vi "Initialize.vi"(8 "error in (no error)":errorcluster, 10 "Laser Configuration":T1, 11 "Laser in":refnum<class "Laser.lvclass">) -> (0 "error out":errorcluster, 3 "Laser out":refnum<class "Laser.lvclass">)   [LabVIEW 2023, in "Laser.lvlib" / "Laser.lvclass"]
uses:
  Laser.lvclass
  Resources/Type Defs/Laser Configuration.ctl
  Laser.lvclass/Laser.ctl
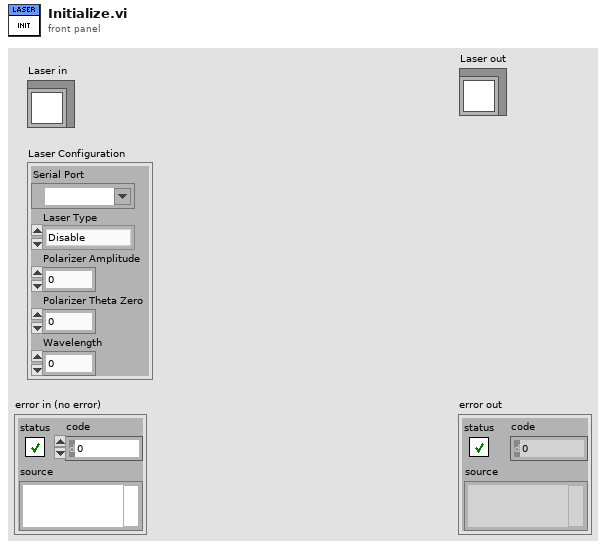
[diagram p1: front panel]
types:
  T1 = typedef "Laser Configuration.ctl" = cluster{"Serial Port":refnum<visa-resource-name>, "Laser Type":enum16{"Disable", "Laser Quantum", "Coherent OBIS", "PRM1-Z8", "Coherent HOPS"}, "Polarizer Amplitude":dbl, "Polarizer Theta Zero":dbl, "Wavelength":u16}
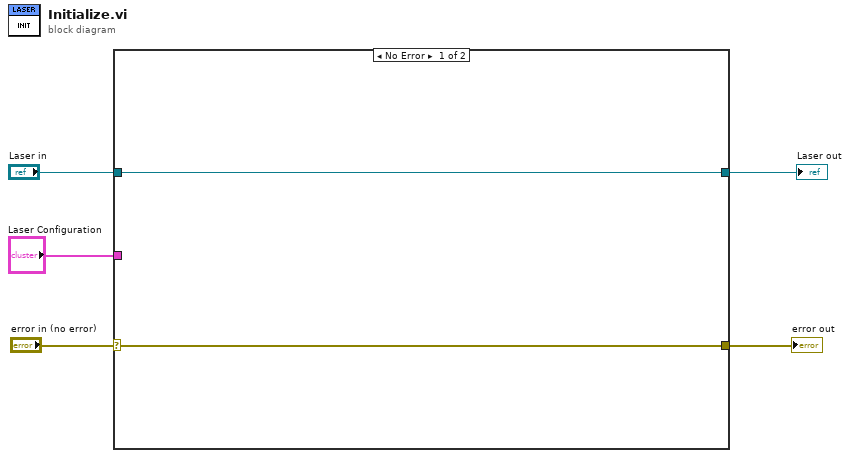
[diagram p0: block diagram]
diagram:
  n1 = case shown="No Error" "error in (no error)" {
    selector: "error in (no error)" -> [w6 w8]
    tunnel: [w7 w9] -> w5
    tunnel: [w6 w8] -> w4
    tunnel: "Laser in" -> [w7 w9]
    tunnel: "Laser Configuration" -> [_ _]
    frame No Error {
    }
    frame Error {
    }
  }
  "error out" <- w4
  "Laser out" <- w5
